vi "Test no error 1097.vi"() -> ()   [LabVIEW 2017, in "unit_tests.lvlib"]
uses:
  unit_tests.lvlib
  libssh2/libssh2_init_default.vi
  libssh2/libssh2.lvlib
  <vilib>/PNR/Transparent Assertions/Transparent Assertions/Transparent Assertions.lvlib
panel:
  out "error out":errorcluster
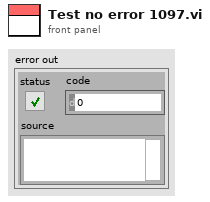
[diagram p1: front panel]
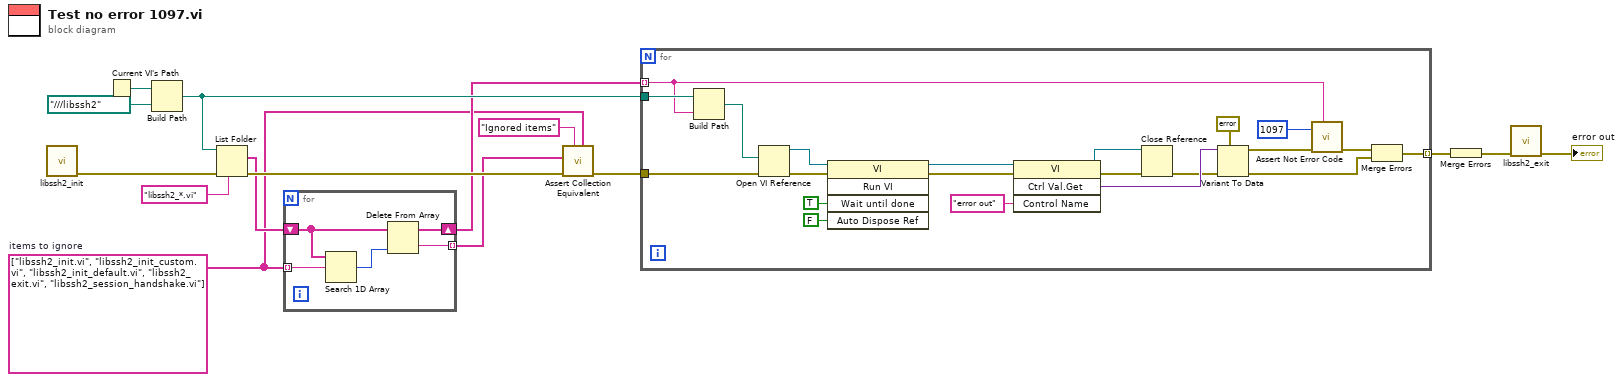
[diagram p0: block diagram]
diagram:
  w3 = string[] ["libssh2_init.vi", "libssh2_init_custom.vi", "libssh2_init_default.vi", "libssh2_exit.vi", "libssh2_session_handshake.vi"]  # items to ignore
  n1 = call-poly "libssh2_init.vi"() -> ("error out"=w9:errorcluster)  [unwired: 11 in]
  n2 = Current VI's Path() -> (path=w15:path)
  n3 = Build Path(base path=w15, name or relative path=path "../../../libssh2" ("base path")) -> (appended path=w12:path)
  n4 = List Folder(path=w12, pattern="libssh2_*.vi", error in=w9) -> (filenames=w6:string[], error out=w10:errorcluster)  [unwired: 1 in, 2 out]
  n5 = for {
    shift-right: [w18] -> w5
    shift-left: w6 -> [w19]
    tunnel: w3 -> [w20] mode=indexing
    tunnel: [w16] -> w2 mode=indexing
    n6 = Search 1D Array(1D array=w19, element=w20) -> (index of element=w17:i32)  [unwired: 1 in]
    n7 = Delete From Array(array=w19, index=w17) -> (deleted portion=w16:string, array with subset deleted=w18:string[])  [unwired: 1 in]
  }
  n8 = call <vilib>:"Assert Collection Equivalent.vi"("Expected"=w3, "Message (\"\")"="Ignored items" ("Label"), "error in (no error)"=w10, "Collection"=w2) -> ("error out"=w4:errorcluster)  [unwired: 7 in]
  n9 = for {
    tunnel: w12 -> [w41]
    tunnel: [w21] -> w11 mode=indexing
    tunnel: w4 -> [w29]
    tunnel: w5 -> [w26] mode=indexing
    n10 = Build Path(base path=w41, name or relative path=w26) -> (appended path=w40:path)
    n11 = Open VI Reference(vi path=w40, error in (no error)=w29) -> (vi reference=w39:refnum<vi>, error out=w35:errorcluster)  [unwired: 4 in]
    n12 = invoke on="Invoke Node" class="VI" method="Run VI"(reference=w39, error in=w35, "Wait until done"=TRUE ("Wait Until Done"), "Auto Dispose Ref"=FALSE ("Auto Dispose Reference")) -> (reference out=w38:refnum<vi>, error out=w34:errorcluster)  [unwired: 1 in, 3 out]
    n13 = invoke on="Invoke Node" class="VI" method="Ctrl Val.Get"(reference=w38, error in=w34, "Control Name"="error out") -> (reference out=w27:refnum<vi>, error out=w32:errorcluster, "Get Control Value Variant"=w31:variant)  [unwired: 1 in, 1 out]
    n14 = Close Reference(reference=w27, error in (no error)=w32) -> (error out=w28:errorcluster)
    n15 = Variant To Data(error in=w28, type=errorcluster {"status"=FALSE, "code"=0, "source"=""} ("error in (no error)"), Variant=w31) -> (data=w23:errorcluster, error out=w22:errorcluster)
    n16 = call <vilib>:"Assert Not Error Code.vi"("Expected"=1097 ("code"), "Message (\"\")"=w26, "error in (no error)"=w23) -> ("error out"=w24:errorcluster)  [unwired: 8 in]
    n17 = Merge Errors(w24, w22) -> (w21:errorcluster)
  }
  n18 = Merge Errors(w11) -> (w7:errorcluster)
  n19 = call "libssh2_exit.vi"("error in (no error)"=w7) -> ("error out"=→"error out":errorcluster)  [unwired: 10 in]
